vi "MakeHTMLParagraph.vi"(3 "Escape Contents":bool, 4 "Paragraph Content":string) -> (1 "Paragraph Element":string)   [LabVIEW 2017, in "ArgosLib.lvlib"]
uses:
  ArgosLib.lvlib
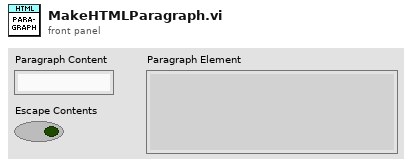
[diagram p1: front panel]
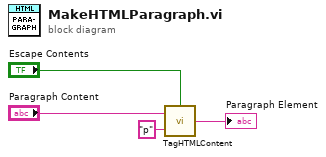
[diagram p0: block diagram]
diagram:
  n1 = call "TagHTMLContent.vi"("Escape Contents"="Escape Contents", "Tag"="p", "Element Contents"="Paragraph Content") -> ("Tagged Contents"=→"Paragraph Element":string)
